vi "State_Machine.vi"(8 "error in (no error)":errorcluster caption="entrée d'erreur (pas d'erreur)", 11 "Get_Voltage en entrée":refnum<class "Nodon_Reset_Voltage_Calibration.lvclass">) -> (0 "error out":errorcluster caption="sortie d'erreur", 2 "Json_String":string, 3 "Get_Voltage en sortie":refnum<class "Nodon_Reset_Voltage_Calibration.lvclass">)   [LabVIEW 2020, in "Library Test.lvlib" / "Nodon_Reset_Voltage_Calibration.lvclass"]
uses:
  Nodon_Reset_Voltage_Calibration.lvclass
  Commun VI/TypeDef/Variable Printable.ctl
  Nodon_Set_Voltage_Calibration/Nodon_Set_Voltage_Calibration.lvclass
  Commun VI/Library Commun.lvlib
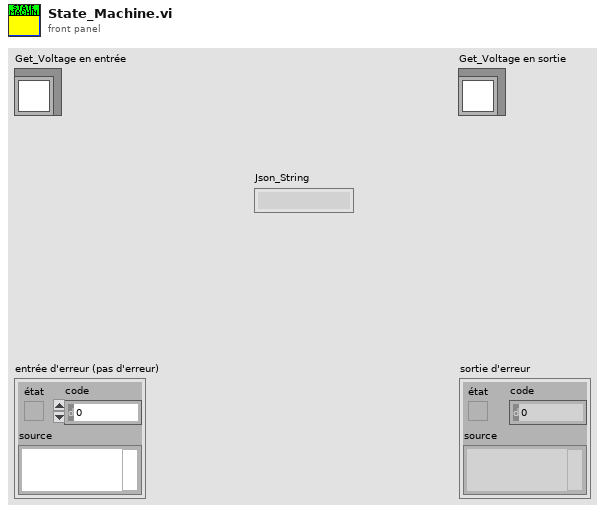
[diagram p1: front panel]
types:
  T1 = typedef "Variable Printable.ctl" = string
  T2 = enum16{"Get Variable", "Get All Variables", "Set Variable", "Delete Variable", "Delete All Variable"}
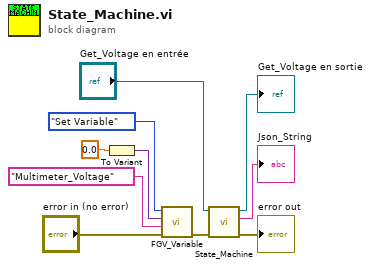
[diagram p0: block diagram]
diagram:
  n1 = To Variant(anything=0.0) -> (Variant=w2:variant)
  n2 = call "FGV_Variable.vi"("error in (no error)"="error in (no error)", "Variable"=T1 "Multimeter_Voltage", "Data In"=w2, "Function"=T2."Set Variable") -> ("error out"=w4:errorcluster)  [unwired: 5 in, 2 out]
  n3 = call-parent "State_Machine.vi"("error in (no error)"=w4, "Get_Voltage en entrée"="Get_Voltage en entrée") -> ("error out"=→"error out":errorcluster, "Json_String"=→"Json_String":string, "Get_Voltage en sortie"=→"Get_Voltage en sortie":refnum<class "Nodon_Reset_Voltage_Calibration.lvclass">)  [unwired: 7 in]
